vi "PZCGetPos.vi"(0 "error in":errorcluster, 1 "Instrument Channel":string="GPIB/0:4,0") -> (2 "Instrument Channel Out":string="GPIB/0:4,0", 3 "Position":i32, 4 "error out":errorcluster)   [LabVIEW 2019]
panel:
  out "Response":string
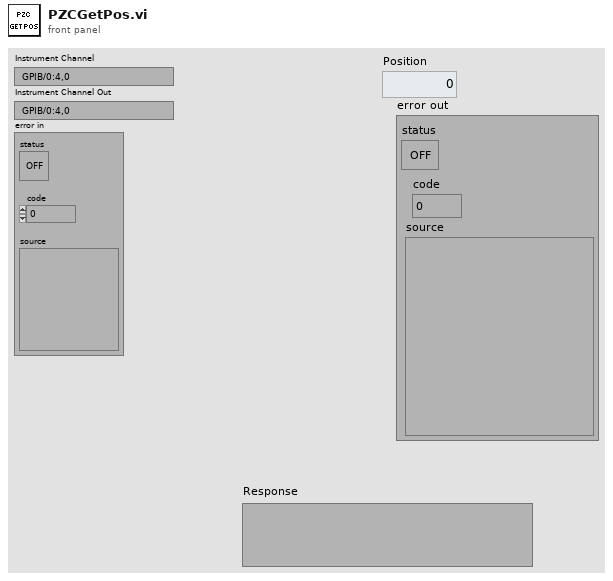
[diagram p1: front panel]
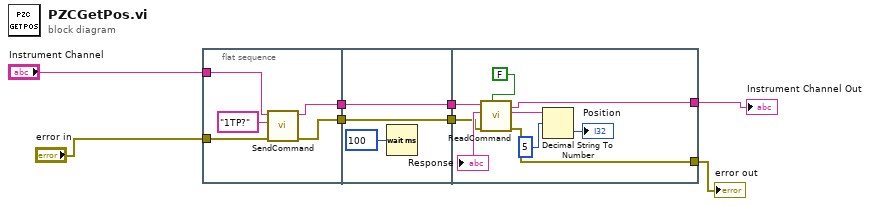
[diagram p0: block diagram]
diagram:
  n1 = flat-sequence {
    tunnel: "Instrument Channel" -> [w12]
    tunnel: [w11] -> w6
    tunnel: [w10] -> w5
    tunnel: "error in" -> [w9]
    tunnel: [w15] -> w7
    tunnel: w6 -> [w15]
    tunnel: w5 -> [w14]
    tunnel: [w14] -> w4
    tunnel: w7 -> [w21]
    tunnel: w4 -> [w20]
    tunnel: [w19] -> w3
    tunnel: [w18] -> w1
    frame #0 {
      n2 = call "SendCommand.vi"("error in"=w9, "Command"="1TP?", "Instrument Channel"=w12) -> ("error out"=w10:errorcluster, "Instrument Channel out"=w11:string)  [unwired: 7 in]
    }
    frame #1 {
      n3 = Wait (ms)(milliseconds to wait=u32 100) -> ()  [unwired: 1 out]
    }
    frame #2 {
      n4 = call "ReadCommand.vi"("Disable MAV check (F)"=FALSE, "error in"=w20, "Instrument Channel"=w21) -> ("error out"=w18:errorcluster, "Response"=w23:string, "Instrument Channel out"=w19:string)  [unwired: 6 in]
      "Response" <- w23
      n5 = Decimal String To Number(string=w23, offset=5) -> (number=→"Position":i32)  [unwired: 1 in, 1 out]
    }
  }
  "Instrument Channel Out" <- w3
  "error out" <- w1
